vi "UT70B read.vi"(11 "string in":string) -> (3 "string out":string)   [LabVIEW 2010]
panel:
  in  "buffer size":u16=22
  in  "baud rate":u32=2400
  in  "data bits":u16=7 min=5 max=8 step=1
  in  "stop bits":enum16{"1 bit", "1.5 bits", "2 bits"}(ring)=enum."2 bits"
  in  "parity":T1(ring)
  in  "port number":i32
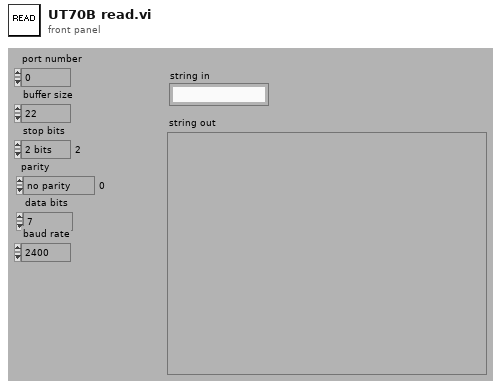
[diagram p1: front panel]
types:
  T1 = enum16{"no parity", "odd parity", "even parity", "mark parity", "space parity"}
  T2 = enum16{"noop", "clear DTR", "set DTR", "clear RTS", "set RTS", "set DTR protocol", "clr DTR protocol", "noop2"}
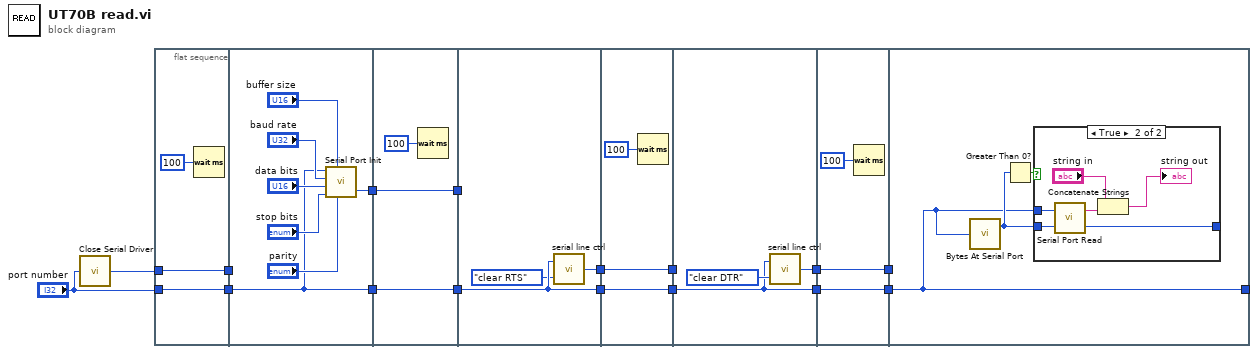
[diagram p0: block diagram]
diagram:
  n1 = call <vilib>:"Close Serial Driver.vi"("port number"="port number") -> ("error"=w2:i32)
  n2 = flat-sequence {
    tunnel: w2 -> [w18]
    tunnel: "port number" -> [w19]
    tunnel: [w19] -> w16
    tunnel: [w18] -> w15
    tunnel: [w21] -> w14
    tunnel: [w20] -> w13
    tunnel: w16 -> [w21]
    tunnel: w15 -> [_]
    tunnel: w14 -> [w29]
    tunnel: [w29] -> w12
    tunnel: w13 -> [w28]
    tunnel: [w28] -> w11
    tunnel: w12 -> [w32]
    tunnel: [w32] -> w10
    tunnel: w11 -> [_]
    tunnel: [w31] -> w9
    tunnel: w10 -> [w35]
    tunnel: [w35] -> w8
    tunnel: w9 -> [w34]
    tunnel: [w34] -> w7
    tunnel: w8 -> [w37]
    tunnel: [w37] -> w6
    tunnel: w7 -> [_]
    tunnel: [w36] -> w5
    tunnel: w6 -> [w41]
    tunnel: [w41] -> w4
    tunnel: w5 -> [w40]
    tunnel: [w40] -> w3
    tunnel: w4 -> [w42]
    tunnel: w3 -> [_]
    tunnel: [w42] -> _
    frame #0 {
      n3 = Wait (ms)(milliseconds to wait=u32 100) -> ()  [unwired: 1 out]
    }
    frame #1 {
      n4 = call <vilib>:"Serial Port Init.vi"("parity"="parity", "buffer size"="buffer size", "stop bits"="stop bits", "data bits"="data bits", "baud rate"="baud rate", "port number"=w21) -> ("error code"=w20:i32)  [unwired: 1 in]
    }
    frame #2 {
      n5 = Wait (ms)(milliseconds to wait=u32 100) -> ()  [unwired: 1 out]
    }
    frame #3 {
      n6 = call <vilib>:"serial line ctrl.vi"("function"=T2."clear RTS", "port number"=w32) -> ("error code"=w31:i32)
    }
    frame #4 {
      n7 = Wait (ms)(milliseconds to wait=u32 100) -> ()  [unwired: 1 out]
    }
    frame #5 {
      n8 = call <vilib>:"serial line ctrl.vi"("function"=T2."clear DTR", "port number"=w37) -> ("error code"=w36:i32)
    }
    frame #6 {
      n9 = Wait (ms)(milliseconds to wait=u32 100) -> ()  [unwired: 1 out]
    }
    frame #7 {
      n10 = call <vilib>:"Bytes At Serial Port.vi"("port number"=w42) -> ("byte count"=w44:u32)  [unwired: 1 out]
      n11 = Greater Than 0?(x=w44) -> (x > 0?=w43:bool)
      n12 = case shown="True" w43 {
        tunnel: w42 -> [_ w49]
        tunnel: w44 -> [w45 w48]
        tunnel: [w45 w47] -> _
        frame False {
        }
        frame True {
          n13 = call <vilib>:"Serial Port Read.vi"("requested byte count"=w48, "port number"=w49) -> ("error code"=w47:i32, "string read"=w51:string)
          n14 = Concatenate Strings("string in", w51) -> (→"string out":string)
        }
      }
    }
  }
